vi "UsrProfiles-Default profile.vi"(8 "error in (no error)":errorcluster) -> (0 "error out":errorcluster, 1 "Selected profile's name":string, 3 "Default profile selected":bool)   [LabVIEW 2020]
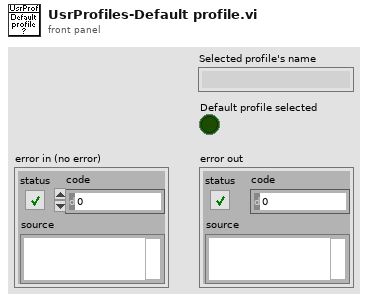
[diagram p1: front panel]
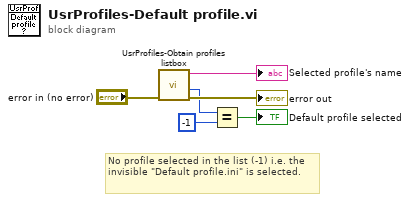
[diagram p0: block diagram]
diagram:
  # "No profile selected in the list (-1) i.e. the invisible \"Default profile.ini\" is selected."
  n1 = call "UsrProfiles-Obtain profiles listbox.vi"("error in (no error)"="error in (no error)") -> ("error out"=→"error out":errorcluster, "Selection's index"=w4:i32, "Selected profile's name"=→"Selected profile's name":string)  [unwired: 7 in, 1 out]
  n2 = Equal?(x=w4, y=-1) -> (x = y?=→"Default profile selected":bool)
